vi "Get Variables.vi"(8 "error in (no error)":errorcluster, 11 "Message Popup in":refnum<class "Timing Functions.lvclass">) -> (0 "error out":errorcluster, 2 "Variables":variant, 3 "Message Popup out":refnum<class "Timing Functions.lvclass">)   [LabVIEW 2016, in "Timing Functions.lvclass"]
uses:
  Timing Functions.lvclass
  Timing Functions.lvclass/Timing Functions.ctl
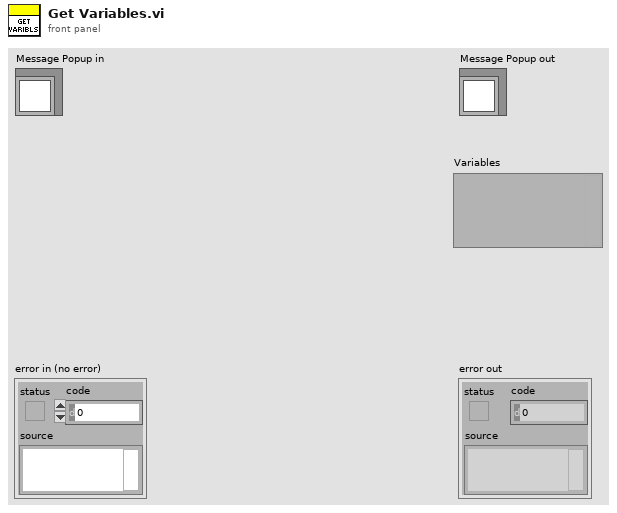
[diagram p1: front panel]
types:
  T1 = typedef "Timing Functions.lvclass/Variables.ctl" = cluster{"seconds":dbl}
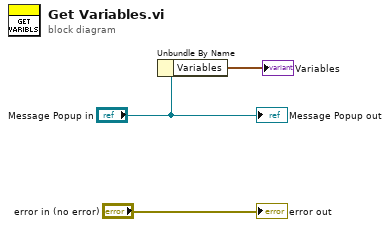
[diagram p0: block diagram]
diagram:
  n1 = Unbundle By Name("Message Popup in") -> ("Variables"=→"Variables":T1)
  "error out" <- "error in (no error)"
  "Message Popup out" <- "Message Popup in"
